vi "Force Icon Editor to Unload.vi"() -> ()   [LabVIEW 2020]
panel:
  out "name found in memory":string
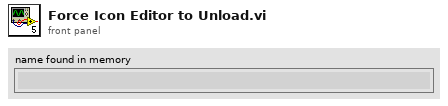
[diagram p1: front panel]
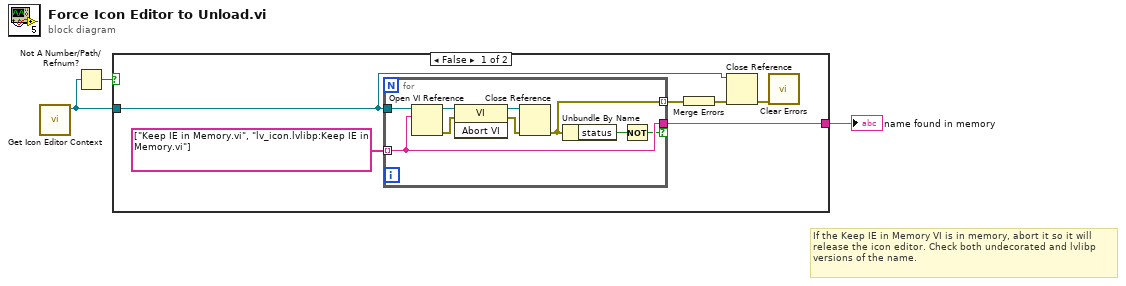
[diagram p0: block diagram]
diagram:
  # "If the Keep IE in Memory VI is in memory, abort it so it will release the icon editor. Check both undecorated and lvlibp versions of the name."
  n1 = call "Get Icon Editor Context.vi"() -> ("icon editor context"=w2:refnum<vi>)  [unwired: 11 in]
  n2 = Not A Number/Path/Refnum?(number/path/refnum=w2) -> (NaN/Path/Refnum?=w1:bool)
  n3 = case shown="False" w1 {
    tunnel: w2 -> [w6 _]
    tunnel: [w7 _] -> w3
    frame False {
      n4 = for {
        tunnel: w6 -> [w17]
        tunnel: string[] ["Keep IE in Memory.vi", "lv_icon.lvlibp:Keep IE in Memory.vi"] -> [w13] mode=indexing
        tunnel: [w12] -> w9 mode=indexing
        tunnel: [w13] -> w7 if=w10
        n5 = Open VI Reference(application reference (local)=w17, vi path=w13) -> (vi reference=w18:refnum<vi>, error out=w14:errorcluster)  [unwired: 1 in, 3 out]
        n6 = invoke class="VI" method="Abort VI"(reference=w18, error in=w14) -> (reference out=w16:refnum<vi>, error out=w15:errorcluster)  [unwired: 1 in, 1 out]
        n7 = Close Reference(reference=w16, error in (no error)=w15) -> (error out=w12:errorcluster)
        n8 = Unbundle By Name(w12) -> ("status"=w11:bool)
        n9 = Not(x=w11) -> (.not. x?=w10:bool)
      }
      n10 = Merge Errors(w9) -> (w4:errorcluster)
      n11 = Close Reference(reference=w6, error in (no error)=w4) -> (error out=w5:errorcluster)
      n12 = call <vilib>:"Clear Errors.vi"("error in (no error)"=w5) -> ()  [unwired: 5 in, 2 out]
    }
    frame True {
    }
  }
  "name found in memory" <- w3
